vi "Pulse Attribute, Calculate Trigger Threshold.vi"(4 "pulse amp":dbl[unit]=-2.3038735826160917 format="%.4f", 5 "error in":errorcluster) -> (0 "error out":errorcluster, 2 "trigger level (V)":dbl=nan format="%.4f")   [LabVIEW 2010]
doc: "This function calculates the trigger level for Pulse Width (Pulse Duration) and Interphase Delay measurements.\n\nIf \"error in\" is TRUE, then \"trigger level (V)\" is set to NaN."
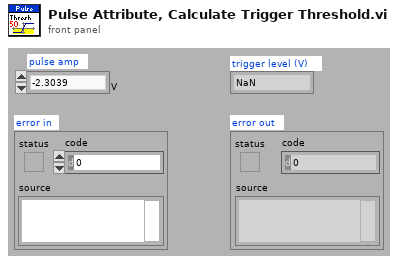
[diagram p1: front panel]
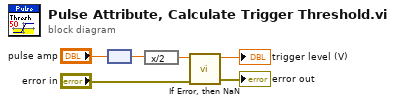
[diagram p0: block diagram]
diagram:
  n1 = node("pulse amp") -> (w1:dbl)
  n2 = expression code="x/2"(w1) -> (w3:dbl)
  n3 = call "If Error, then NaN.vi"("error in (T)"="error in", "value1"=w3) -> ("error out"=→"error out":errorcluster, "value out1"=→"trigger level (V)":dbl)  [unwired: 4 in, 2 out]
